vi "test_LogSink_LogManyEvents_AllEventsCaptured.vi"(8 "error in (no error)":errorcluster, 11 "TestCase in":refnum<class "TestDataSink.lvclass">) -> (0 "error out":errorcluster, 3 "TestCase out":refnum<class "TestDataSink.lvclass">)   [LabVIEW 2017, in "TestDataSink.lvclass"]
uses:
  TestDataSink.lvclass
  Source/Composed Log/Types/Log Level.ctl
  Source/Composed Log/LoggerReference/LoggerReference.lvclass/LoggerReference.ctl
  Source/LVQueue Sink/LVQueue Sink.lvclass/LVQueue Sink.ctl
  9102acfd-f255-4d38-bc0e-2cbfe0040564.vi
  9102acfd-f255-4d38-bc0e-2cbfe0040564.vi/eaf86a5d-0de1-4b6c-9a9d-50b4ebb37b3b.vi
  Source/Composed Log/LoggerReference/Return Aggregate Queues.vi
  Source/Composed Log/LoggerReference/Add Aggregate Log.vi
  9102acfd-f255-4d38-bc0e-2cbfe0040564.vi/eaf86a5d-0de1-4b6c-9a9d-50b4ebb37b3b.vi/428f1194-cf7f-42d6-b14f-8753ce8757d1.vi
  Source/Composed Log/LoggerReference/Log.vi
  Source/Composed Log/LoggerReference/Send Add Sink.vi
  Source/Composed Log/LoggerReference/Remove Stale Logs.vi
  Source/LVQueue Sink/LVQueue Sink.lvclass
  C:/CS/Internal/LabVIEW/Logger/Source/Composed Log/Log Sink/Log Sink.lvclass
  Source/Composed Log/Application Logger/Launch Worker Loop.vi
  Source/Composed Log/LoggerReference/Initialize Logger Instance.vi
  Source/Composed Log/Singleton Event Log/Logger Queue FGV.vi
  Source/Composed Log/IErrorFormat/IErrorFormat.lvclass
  Source/Composed Log/LoggerReference/LoggerReference.lvclass
  Source/Composed Log/Log Sink/Log Sink.lvclass
  <vilib>/addons/_JKI Toolkits/VI Tester/TestCase.llb/TestCase.lvclass
  Source/Composed Log/Singleton Event Log/Singleton Event Log.lvlib
  Source/Composed Log/Composed Log.lvlib
  C:/Program Files (x86)/National Instruments/LabVIEW 2017/vi.lib/addons/_JKI Toolkits/VI Tester/TestCase.llb/TestCase.lvclass
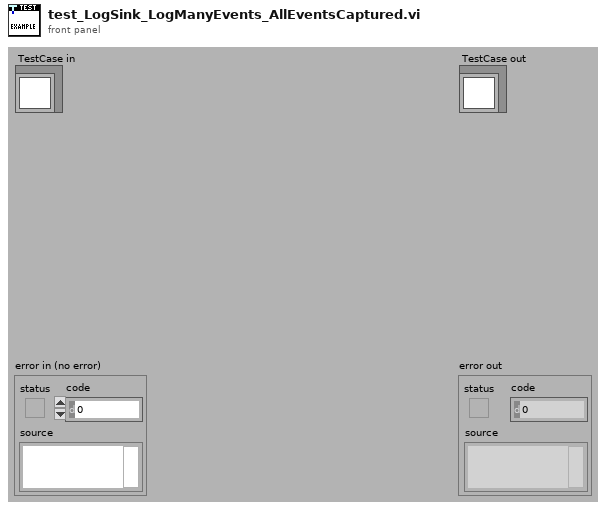
[diagram p1: front panel]
types:
  T1 = typedef "Composed Log.lvlib/Log Level.ctl" = enum16{"Debug", "Info", "Warning", "Error", "Critical"}
  T2 = typedef "Composed Log.lvlib/Log Packet.ctl" = cluster{"Data To Log":string, "Source":string, "Event Level":T1, "Event Time":timestamp}
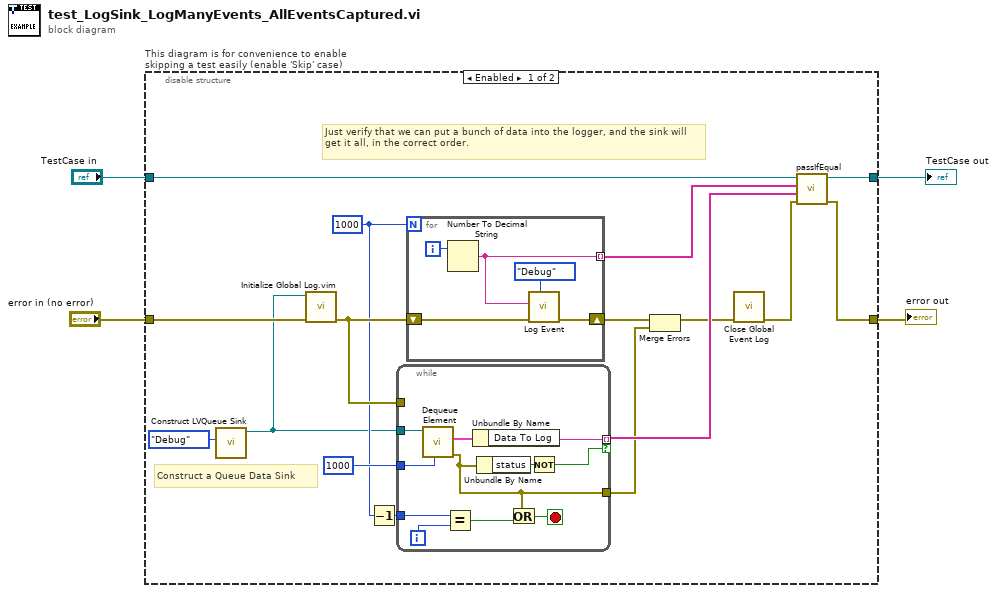
[diagram p0: block diagram]
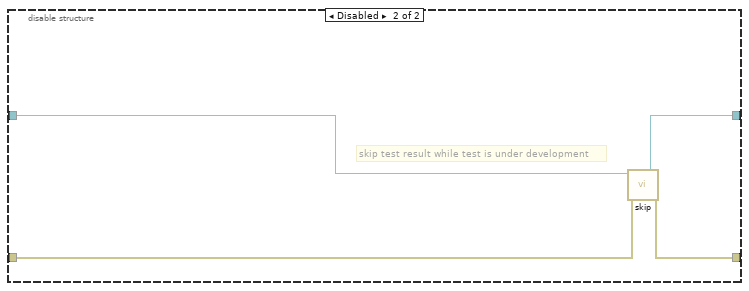
[diagram p2: hidden frame]
diagram:
  n1 = disable-structure "This diagram is for convenience to enable skipping a test easily (enable 'Skip' case)" shown="Enabled" {
    disable-tunnel: "TestCase in" -> [w14 w40]
    disable-tunnel: [w17 w38] -> w1
    disable-tunnel: [w16 w39] -> w3
    disable-tunnel: "error in (no error)" -> [w20 w37]
    frame Enabled {
      w7 = 1000
      # "Just verify that we can put a bunch of data into the logger, and the sink will get it all, in the correct order."
      # "Construct a Queue Data Sink"
      n2 = call "Construct LVQueue Sink.vi"("LogLevel"=Log_Level."Debug") -> ("LVQueue Sink out"=w5:refnum<class "LVQueue Sink.lvclass">)  [unwired: 9 in, 1 out]
      n3 = call "Initialize Global Log.vim"("error in (no error)"=w20, "Log Sink(s)"=w5) -> ("error out"=w12:errorcluster)  [unwired: 8 in, 1 out]
      n4 = Decrement(x=w7) -> (x-1=w6:i32)
      n5 = while {
        tunnel: w5 -> [w31]
        tunnel: [w29] -> w11 mode=indexing if=w28
        tunnel: w12 -> [_]
        tunnel: 1000 ("timeout in ms (-1)") -> [w26]
        tunnel: [w22] -> w8
        tunnel: w6 -> [w24]
        i -> [w25]
        stop <- w21 stop-if-true
        n6 = call "Dequeue Element.vi"("timeout in ms (-1)"=w26, "LVQueue Sink in"=w31) -> ("error out"=w22:errorcluster, "Log Packet"=w30:T2)  [unwired: 6 in, 2 out]
        n7 = Equal?(x=w24, y=w25) -> (x = y?=w23:bool)
        n8 = Unbundle By Name(w30) -> ("Data To Log"=w29:string)
        n9 = Unbundle By Name(w22) -> ("status"=w27:bool)
        n10 = Or(x=w22, y=w23) -> (x .or. y?=w21:bool)
        n11 = Not(x=w27) -> (.not. x?=w28:bool)
      }
      n12 = for {
        N: w7 -> [_]
        shift-right: [w33] -> w18
        shift-left: w12 -> [w35]
        tunnel: [w34] -> w13 mode=indexing
        i -> [w36]
        n13 = Number To Decimal String(number=w36) -> (decimal integer string=w34:string)  [unwired: 1 in]
        n14 = call "Log Event.vi"("Event Level"=Log_Level."Debug", "error in (no error)"=w35, "Data To Log"=w34) -> ("error out"=w33:errorcluster)  [unwired: 8 in]
      }
      n15 = Merge Errors(w18, w8) -> (w9:errorcluster)
      n16 = call "Close Global Event Log.vi"("error in (no error)"=w9) -> ("error out"=w15:errorcluster)  [unwired: 10 in]
      n17 = call-dynamic "passIfEqual.vi"("error in (no error)"=w15, "y"=w11, "x"=w13, "TestCase in"=w14) -> ("error out"=w16:errorcluster, "TestCase out"=w17:refnum<class "TestDataSink.lvclass">)  [unwired: 6 in]
    }
    frame Disabled {
      # "skip test result while test is under development"
      n18 = call <vilib>:"skip.vi"("error in (no error)"=w37, "TestCase in"=w40) -> ("error out"=w39:errorcluster, "TestCase out"=w38:refnum<class "TestDataSink.lvclass">)  [unwired: 8 in]
    }
  }
  "error out" <- w3
  "TestCase out" <- w1
